vi "Mute gRPC Server Common Errors.vi"(8 "error in (no error)":errorcluster, 11 "Errors to Mute":i32[](array[numeric])=[-1001, -2]) -> (0 "error out":errorcluster)   [LabVIEW 2021, in "CIFCorePlugin.lvclass"]
doc: "Mute errors from the gRPC server that are common and don't indicate a core failure. The default errors to clear are from gRPC client timeout and cancel."
uses:
  CIFCorePlugin.lvclass
  CIFCorePlugin.lvclass/CIFCorePlugin.ctl
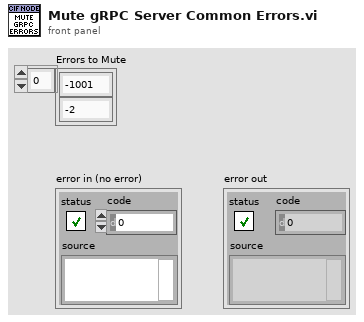
[diagram p1: front panel]
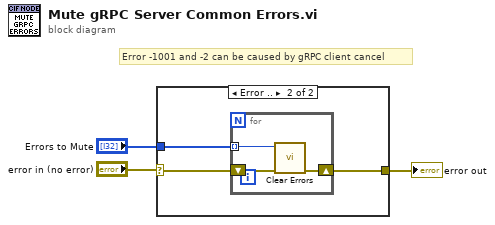
[diagram p0: block diagram]
diagram:
  # "Error -1001 and -2 can be caused by gRPC client cancel"
  n1 = case shown="Error .." "error in (no error)" {
    selector: "error in (no error)" -> [w4 w7]
    tunnel: [w4 w6] -> w2
    tunnel: "Errors to Mute" -> [_ w5]
    frame No Error {
    }
    frame Error {
      n2 = for {
        shift-right: [w9] -> w6
        shift-left: w7 -> [w10]
        tunnel: w5 -> [w8] mode=indexing
        n3 = call <vilib>:"Clear Errors.vi"("error in (no error)"=w10, "specific error code to clear (0: all)"=w8) -> ("error out"=w9:errorcluster)  [unwired: 4 in, 1 out]
      }
    }
  }
  "error out" <- w2
